vi "OperatorControlBox_Joystick_Name.vi"(3 "POVs":i16[](array[numeric]), 4 "Buttons":bool[](array[boolean]), 5 "Axes":dbl[](array[numeric])) -> (0 "Connected":bool, 1 "Named Buttons":T1)   [LabVIEW 2018]
uses:
  TypeDefs/OperatorControlBoxButtons_Type.ctl
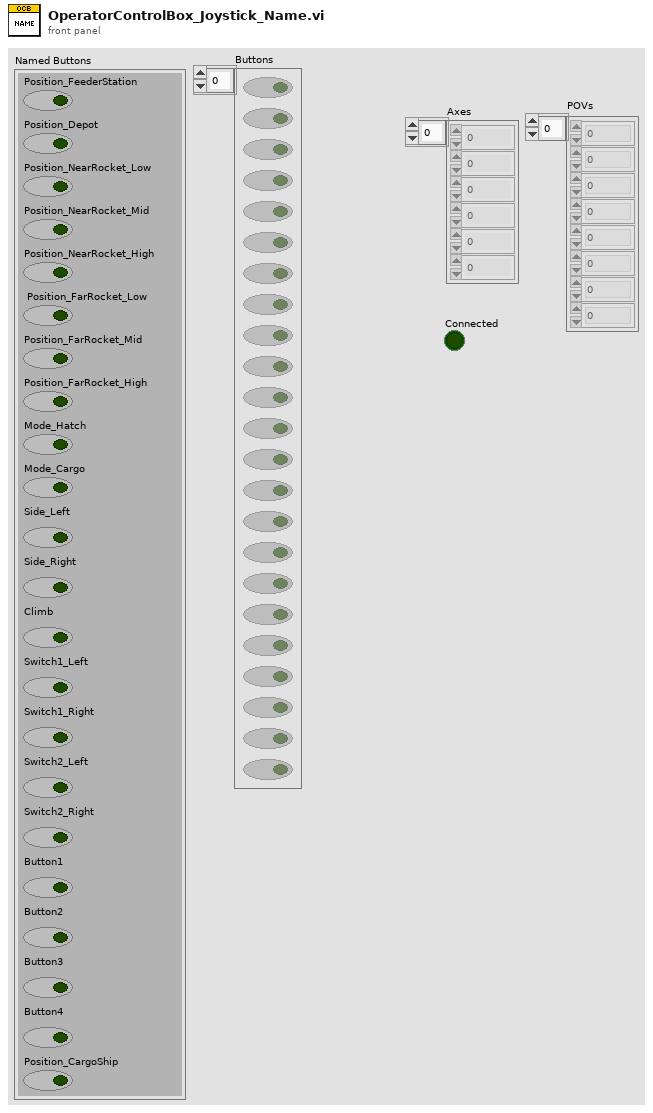
[diagram p1: front panel]
types:
  T1 = typedef "OperatorControlBoxButtons_Type.ctl" = cluster{"Position_FeederStation":bool, "Position_Depot":bool, "Position_NearRocket_Low":bool, "Position_NearRocket_Mid":bool, "Position_NearRocket_High":bool, " Position_FarRocket_Low":bool, "Position_FarRocket_Mid":bool, "Position_FarRocket_High":bool, "Mode_Hatch":bool, "Mode_Cargo":bool, "Side_Left":bool, "Side_Right":bool, "Climb":bool, "Switch1_Left":bool, "Switch1_Right":bool, "Switch2_Left":bool, "Switch2_Right":bool, "Button1":bool, "Button2":bool, "Button3":bool, "Button4":bool, "Position_CargoShip":bool}
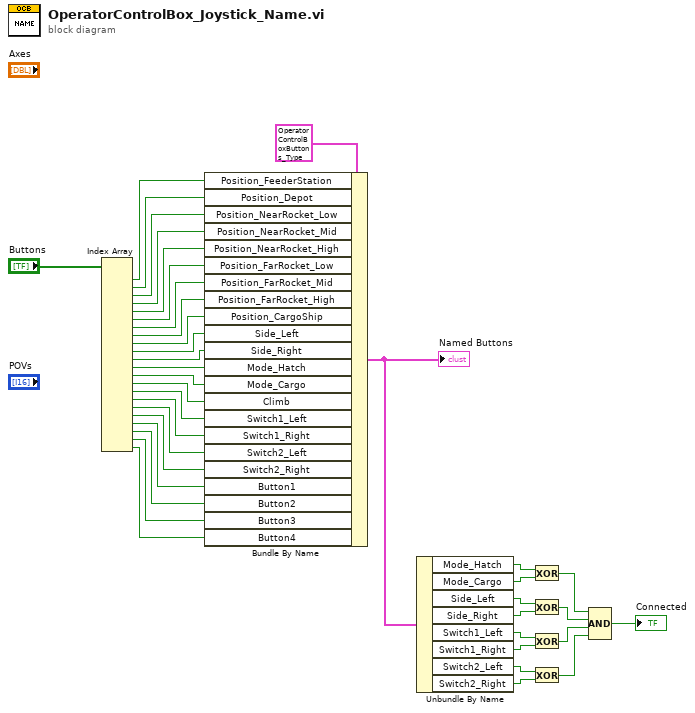
[diagram p0: block diagram]
diagram:
  n1 = Index Array(array="Buttons") -> (element #1=w37:bool, element #2=w36:bool, element #3=w35:bool, element #4=w34:bool, element #5=w33:bool, element #6=w32:bool, element #7=w31:bool, element #8=w30:bool, element #9=w29:bool, element #10=w28:bool, element #11=w27:bool, element #12=w26:bool, element #13=w25:bool, element #14=w24:bool, element #15=w23:bool, element #16=w22:bool, element #17=w21:bool, element #18=w20:bool, element #19=w19:bool, element #20=w18:bool, element #21=w17:bool, element #22=w16:bool)  [unwired: 22 in]
  n2 = Bundle By Name(cluster=T1 {"Position_FeederStation"=FALSE, "Position_Depot"=FALSE, "Position_NearRocket_Low"=FALSE, "Position_NearRocket_Mid"=FALSE, "Position_NearRocket_High"=FALSE, " Position_FarRocket_Low"=FALSE, "Position_FarRocket_Mid"=FALSE, "Position_FarRocket_High"=FALSE, "Mode_Hatch"=FALSE, "Mode_Cargo"=FALSE, "Side_Left"=FALSE, "Side_Right"=FALSE, "Climb"=FALSE, "Switch1_Left"=FALSE, "Switch1_Right"=FALSE, "Switch2_Left"=FALSE, "Switch2_Right"=FALSE, "Button1"=FALSE, "Button2"=FALSE, "Button3"=FALSE, "Button4"=FALSE, "Position_CargoShip"=FALSE}, "Position_FeederStation"=w37, "Position_Depot"=w36, "Position_NearRocket_Low"=w35, "Position_NearRocket_Mid"=w34, "Position_NearRocket_High"=w33, "Position_FarRocket_Low"=w32, "Position_FarRocket_Mid"=w31, "Position_FarRocket_High"=w30, "Position_CargoShip"=w29, "Side_Left"=w28, "Side_Right"=w27, "Mode_Hatch"=w26, "Mode_Cargo"=w25, "Climb"=w24, "Switch1_Left"=w23, "Switch1_Right"=w22, "Switch2_Left"=w21, "Switch2_Right"=w20, "Button1"=w19, "Button2"=w18, "Button3"=w17, "Button4"=w16) -> (w14:T1)
  "Named Buttons" <- w14
  n3 = Unbundle By Name(w14) -> ("Mode_Hatch"=w12:bool, "Mode_Cargo"=w13:bool, "Side_Left"=w11:bool, "Side_Right"=w10:bool, "Switch1_Left"=w9:bool, "Switch1_Right"=w8:bool, "Switch2_Left"=w7:bool, "Switch2_Right"=w6:bool)
  n4 = Exclusive Or(1:w13, 2:w12) -> (0:w2:bool)
  n5 = Exclusive Or(1:w10, 2:w11) -> (0:w5:bool)
  n6 = Exclusive Or(1:w8, 2:w9) -> (0:w4:bool)
  n7 = Exclusive Or(1:w6, 2:w7) -> (0:w3:bool)
  n8 = Compound Arithmetic op=AND(w2, w5, w4, w3) -> (→"Connected":bool)
